vi "myProgram.vi"() -> ()   [LabVIEW 2019]
uses:
  <vilib>/numeric/Random Number (Range) I64.vi
  <vilib>/numeric/sub_Random U32.vi
panel:
  out "String":string
  out "Boolean 2":bool
  in  "Boolean":bool
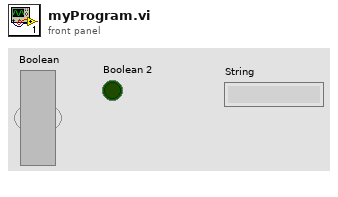
[diagram p1: front panel]
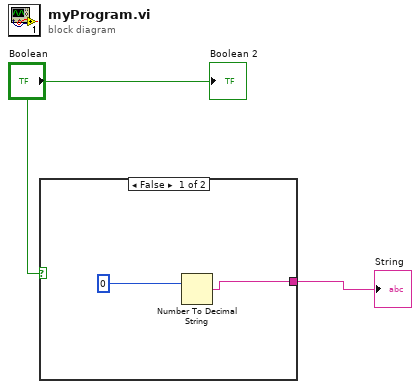
[diagram p0: block diagram]
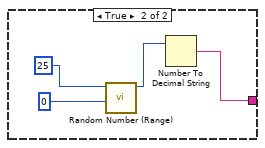
[diagram p2: hidden frame]
diagram:
  n1 = case shown="False" "Boolean" {
    tunnel: [w3 w5] -> w2
    frame False {
      n2 = Number To Decimal String(number=0) -> (decimal integer string=w3:string)  [unwired: 1 in]
    }
    frame True {
      n3 = call-poly <vilib>:"Random Number (Range).vi"("lower bound (-100)"=0, "upper bound (100)"=25) -> ("number"=w8:i64)  [unwired: 9 in]
      n4 = Number To Decimal String(number=w8) -> (decimal integer string=w5:string)  [unwired: 1 in]
    }
  }
  "String" <- w2
  "Boolean 2" <- "Boolean"
